vi "MT method (SubVI).vi"(0 "Shift Register in 1":u32 format="%#_6f", 1 "Encoder pulses":i32 format="%#_6f", 2 "Tick Count (mSec)":u32 format="%#_6f", 3 "Tc (mSec)":u32 format="%#_6f", 5 "Shift Register in 2":i32 format="%#_6f", 7 "Shift Register in 3":i32 format="%#_6f", 9 "m1_pre":i32 format="%#_6f", 11 "m2_pre":u32 format="%#_6f") -> (4 "Shift Register out 1":u32 format="%#_6f", 6 "Shift Register out 2":i32 format="%#_6f", 8 "Shift Register out 3":i32 format="%#_6f", 10 "m1":i32 format="%#_6f", 15 "m2":u32 format="%#_6f")   [LabVIEW 2014]
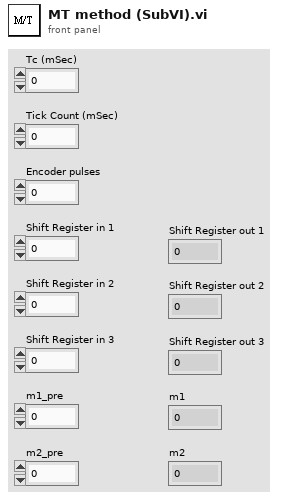
[diagram p1: front panel]
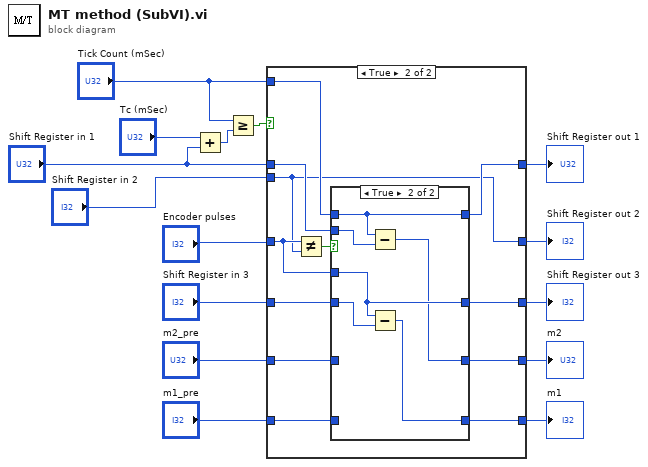
[diagram p0: block diagram]
diagram:
  n1 = Add(x="Tc (mSec)", y="Shift Register in 1") -> (x+y=w6:u32)
  n2 = Greater Or Equal?(x="Tick Count (mSec)", y=w6) -> (x >= y?=w5:bool)
  n3 = case shown="True" w5 {
    tunnel: [w20 w32] -> w7
    tunnel: "Tick Count (mSec)" -> [_ w31]
    tunnel: "Shift Register in 1" -> [w20 w30]
    tunnel: [w19 w25] -> w10
    tunnel: "Encoder pulses" -> [w19 w26]
    tunnel: "Shift Register in 2" -> [_ w25]
    tunnel: [w18 w28] -> w13
    tunnel: "Shift Register in 3" -> [w18 w27]
    tunnel: [w17 w24] -> w4
    tunnel: [w16 w23] -> w3
    tunnel: "m2_pre" -> [w17 w22]
    tunnel: "m1_pre" -> [w16 w21]
    frame False {
    }
    frame True {
      n4 = Not Equal?(x=w26, y=w25) -> (x != y?=w29:bool)
      n5 = case shown="True" w29 {
        tunnel: [w36 w42] -> w32
        tunnel: w31 -> [_ w42]
        tunnel: w30 -> [w36 w41]
        tunnel: [w35 w40] -> w28
        tunnel: w27 -> [w35 w39]
        tunnel: w26 -> [_ w40]
        tunnel: [w34 w38] -> w24
        tunnel: [w33 w37] -> w23
        tunnel: w22 -> [w34 _]
        tunnel: w21 -> [w33 _]
        frame False {
        }
        frame True {
          n6 = Subtract(x=w42, y=w41) -> (x-y=w38:u32)
          n7 = Subtract(x=w40, y=w39) -> (x-y=w37:i32)
        }
      }
    }
  }
  "Shift Register out 3" <- w13
  "Shift Register out 2" <- w10
  "Shift Register out 1" <- w7
  "m2" <- w4
  "m1" <- w3
